vi "SubConfocal_DiskSpinningOnOff.vi"(7 "Confocal scanner":T1={"SDC shutter"=FALSE, "Filter wheel"=3, "FW speed"=3, "Disk spinning"=FALSE, "Disk speed (rpm)"=3000.0} {"Disk speed (rpm)" min=1500.0 max=10000.0; "FW speed" min=1 max=5 step=1; "Filter wheel" items=["CFP"=1, "GFP"=2, "mCherry"=3, "Alexa-647"=4, "OFP"=5, "empty"=6]}, 8 "Error In":errorcluster, 11 "Confocal line (VISA IN)":refnum<visa-resource-name>="COM1") -> (0 "Error out":errorcluster, 3 "VISA OUT":refnum<visa-resource-name>="COM1")   [LabVIEW 2015]
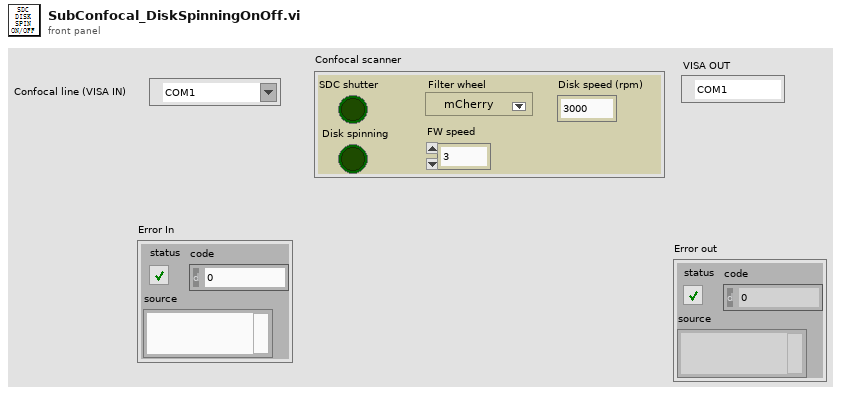
[diagram p1: front panel]
types:
  T1 = cluster{"SDC shutter":bool, "Filter wheel":u16, "FW speed":i32, "Disk spinning":bool, "Disk speed (rpm)":dbl}
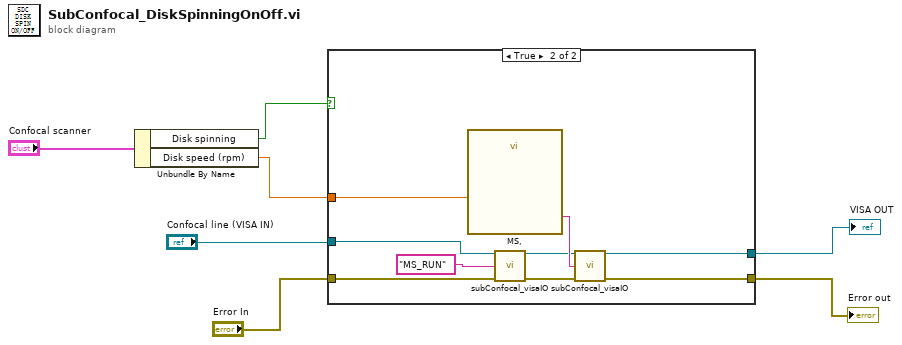
[diagram p0: block diagram]
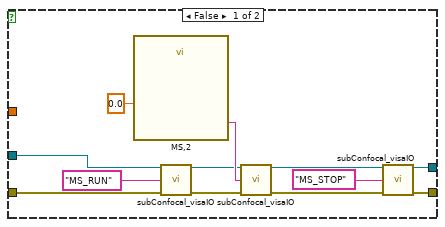
[diagram p2: hidden frame]
diagram:
  n1 = Unbundle By Name("Confocal scanner") -> ("Disk spinning"=w1:bool, "Disk speed (rpm)"=w4:dbl)
  n2 = case shown="True" w1 {
    tunnel: "Confocal line (VISA IN)" -> [w13 w27]
    tunnel: [w18 w24] -> w5
    tunnel: "Error In" -> [w11 w23]
    tunnel: [w17 w21] -> w6
    tunnel: w4 -> [_ w20]
    frame False {
      n3 = call "MS,2"("R"=0.0) -> ("Result"=w15:string)  [unwired: 13 in, 1 out]
      n4 = call "subConfocal_visaIO.vi"("VISA  IN"=w13, "Command (to ctlr)"="MS_RUN", "error in"=w11) -> ("VISA OUT"=w14:refnum<visa-resource-name>, "error out"=w10:errorcluster)  [unwired: 8 in, 3 out]
      n5 = call "subConfocal_visaIO.vi"("VISA  IN"=w14, "Command (to ctlr)"=w15, "error in"=w10) -> ("VISA OUT"=w12:refnum<visa-resource-name>, "error out"=w9:errorcluster)  [unwired: 8 in, 3 out]
      n6 = call "subConfocal_visaIO.vi"("VISA  IN"=w12, "Command (to ctlr)"="MS_STOP", "error in"=w9) -> ("VISA OUT"=w18:refnum<visa-resource-name>, "error out"=w17:errorcluster)  [unwired: 8 in, 3 out]
    }
    frame True {
      n7 = call "MS,"("R"=w20) -> ("Result"=w26:string)  [unwired: 13 in, 1 out]
      n8 = call "subConfocal_visaIO.vi"("VISA  IN"=w27, "Command (to ctlr)"="MS_RUN", "error in"=w23) -> ("VISA OUT"=w25:refnum<visa-resource-name>, "error out"=w22:errorcluster)  [unwired: 8 in, 3 out]
      n9 = call "subConfocal_visaIO.vi"("VISA  IN"=w25, "Command (to ctlr)"=w26, "error in"=w22) -> ("VISA OUT"=w24:refnum<visa-resource-name>, "error out"=w21:errorcluster)  [unwired: 8 in, 3 out]
    }
  }
  "VISA OUT" <- w5
  "Error out" <- w6
